vi "verify acquisition finished SPARC4.vi"(8 "error in (no error)":errorcluster, 11 "Save Image in":refnum<class "Save SPARC4 image.lvclass">) -> (0 "error out":errorcluster, 2 "acq finished":T1, 3 "Save Image out":refnum<class "Save SPARC4 image.lvclass">)   [LabVIEW 2018, in "Save SPARC4 image.lvclass"]
uses:
  Save SPARC4 image.lvclass
  C:/Users/Denis/Desktop/S4ACS/S4ACS/Save Image/Save Image.lvclass
  SPARC4_Channel/SPARC4_Channel.lvclass/SPARC4_Channel.ctl
  SPARC4_Channel/SPARC4_Channel.lvclass
  Save Image/Save Image.lvclass
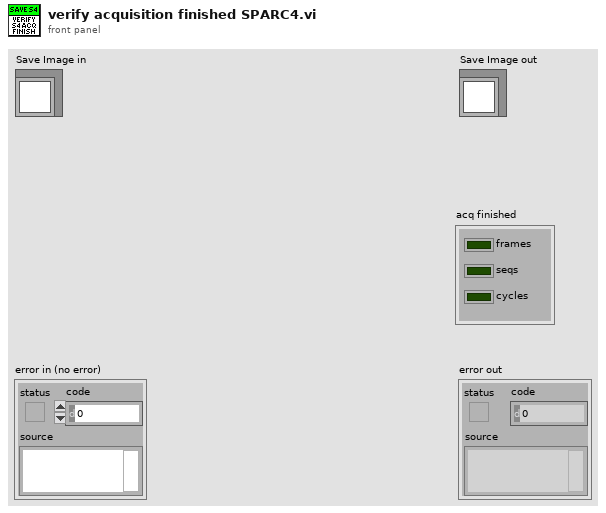
[diagram p1: front panel]
types:
  T1 = cluster{"frames":bool, "seqs":bool, "cycles":bool}
  T2 = cluster{"#SEQS":u32, "WAVEPLATE_POS":i32, "Waveplate positions":u8[]}
  T3 = cluster{"SEQS_DONE":u16, "S4ICS comm attempts":u8}
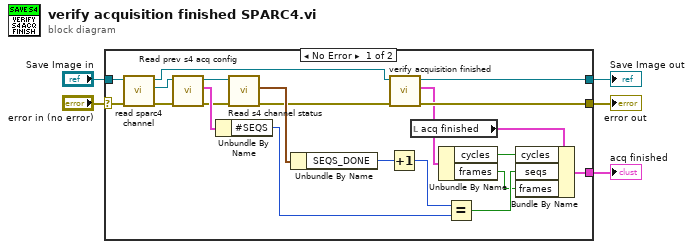
[diagram p0: block diagram]
diagram:
  n1 = case shown="No Error" "error in (no error)" {
    selector: "error in (no error)" -> [w9 w28]
    tunnel: [w14 w28] -> w4
    tunnel: [w15 w27] -> w2
    tunnel: "Save Image in" -> [w10 w27]
    tunnel: [w18 _] -> w1
    frame No Error {
      n2 = call "read sparc4 channel.vi"("error in (no error)"=w9, "Save SPARC4 image in"=w10) -> ("error out"=w6:errorcluster, "sparc4 channel"=w7:refnum<class "SPARC4_Channel.lvclass">, "Save SPARC4 image out"=w8:refnum<class "Save SPARC4 image.lvclass">)  [unwired: 7 in]
      n3 = call "Read prev s4 acq config.vi"("error in (no error)"=w6, "SPARC4_Channel in"=w7) -> ("error out"=w19:errorcluster, "prev s4 acq config"=w22:T2, "SPARC4_Channel out"=w20:refnum<class "SPARC4_Channel.lvclass">)  [unwired: 6 in, 1 out]
      n4 = Unbundle By Name(w22) -> ("#SEQS"=w21:u32)
      n5 = call "Read s4 channel status.vi"("error in (no error)"=w19, "SPARC4_Channel in"=w20) -> ("error out"=w25:errorcluster, "s4 channel status"=w26:T3)  [unwired: 6 in, 2 out]
      n6 = Unbundle By Name(w26) -> ("SEQS_DONE"=w17:u16)
      n7 = Increment(x=w17) -> (x+1=w16:u16)
      n8 = call "verify acquisition finished.vi"("error in (no error)"=w25, "Save Image in"=w8) -> ("error out"=w14:errorcluster, "acq finished"=w13:cluster{"frames":bool, "cycles":bool}, "Save Image out"=w15:refnum<class "Save SPARC4 image.lvclass">)  [unwired: 7 in]
      n9 = local read "acq finished"() -> (w24:T1)
      n10 = Unbundle By Name(w13) -> ("cycles"=w12:bool, "frames"=w11:bool)
      n11 = Equal?(x=w16, y=w21) -> (x = y?=w23:bool)
      n12 = Bundle By Name(cluster=w24, "cycles"=w12, "seqs"=w23, "frames"=w11) -> (w18:T1)
    }
    frame Error {
    }
  }
  "error out" <- w4
  "Save Image out" <- w2
  "acq finished" <- w1
